vi "Calibrate Ticks 2 Speed (uSMC).vi"(2 "speed ticks":u16) -> (0 "speed value (units)":dbl)   [LabVIEW 2010, in "SignalWriterMH110203USBStepperMotor.lvclass"]
uses:
  SignalWriterMH110203USBStepperMotor.lvclass
  class_data.vi
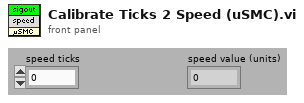
[diagram p1: front panel]
types:
  T1 = typedef "SignalWriterMH110203USBStepperMotor.lvclass/GoTo Control (uSMC).ctl" = cluster{"Step motor ID":string, "SMname":string, "Backlash":u16, "wait for input sygnal to start":bool, "use slow start/stop":bool, "units name":string, "Maximum speed":dbl, "speed":dbl, "step":u8, "point 1 ticks":i32, "point 2 ticks":i32, "point 1 units":dbl, "point 2 units":dbl, "Limit Switch standoff":dbl, "Zero Value":dbl, "Destination Position":dbl, "force backlash":bool, "power off when stop":bool, "POff delay":dbl, "positioner name":string, "R, Ohm":dbl, "I, mA":dbl, "Positioner's Type":u16, "Reset Direction":bool, "Manufacturer":string, "Model":string, "Scheme":string, "FirmwareVer":string}
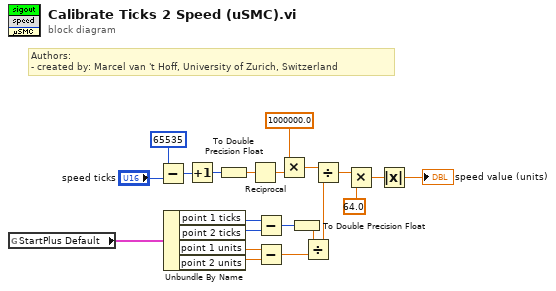
[diagram p0: block diagram]
diagram:
  # "Authors: \n- created by: Marcel van 't Hoff, University of Zurich, Switzerland"
  n1 = global read "class_data.vi" "StartPlus Default"() -> (w1:T1)
  n2 = Subtract(x=u16 65535, y="speed ticks") -> (x-y=w19:u16)
  n3 = Unbundle By Name(w1) -> ("point 1 ticks"=w14:i32, "point 2 ticks"=w13:i32, "point 1 units"=w12:dbl, "point 2 units"=w11:dbl)
  n4 = Increment(x=w19) -> (x+1=w18:u16)
  n5 = To Double Precision Float(number=w18) -> (double precision float=w15:dbl)
  n6 = Reciprocal(x=w15) -> (1/x=w17:dbl)
  n7 = Subtract(x=w14, y=w13) -> (x-y=w9:i32)
  n8 = Subtract(x=w12, y=w11) -> (x-y=w10:dbl)
  n9 = Multiply(x=1000000.0, y=w17) -> (x*y=w5:dbl)
  n10 = To Double Precision Float(number=w9) -> (double precision float=w8:dbl)
  n11 = Divide(x=w8, y=w10) -> (x/y=w7:dbl)
  n12 = Divide(x=w5, y=w7) -> (x/y=w6:dbl)
  n13 = Multiply(x=w6, y=64.0 ("x")) -> (x*y=w4:dbl)
  n14 = Absolute Value(x=w4) -> (abs(x)=→"speed value (units)":dbl)
